vi "SetTrigger.vi"(8 "error in (no error)":errorcluster, 10 "Settings.Trigger":T1, 11 "ThorLabsCsCamera in":refnum<class "ThorLabsCsCamera.lvclass">) -> (0 "error out":errorcluster, 2 "Settings.Trigger  out":T1, 3 "ThorLabsCsCamera out":refnum<class "ThorLabsCsCamera.lvclass">)   [LabVIEW 2020, in "ThorLabsCsCamera.lvclass"]
uses:
  ThorLabsCsCamera.lvclass
  OnOffTypeDef.ctl
  ThorLabsCsCamera.lvclass/ThorLabsCsCamera.ctl
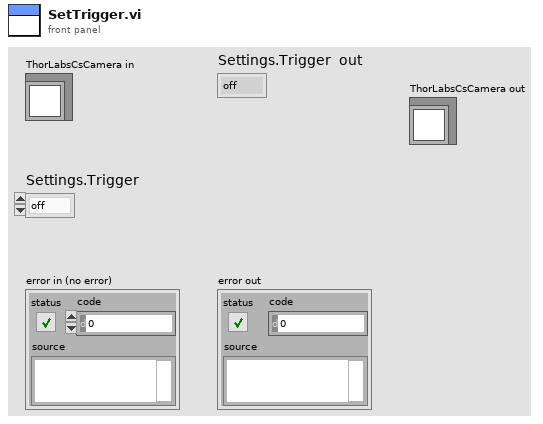
[diagram p1: front panel]
types:
  T1 = typedef "OnOffTypeDef.ctl" = enum16{"off", "on"}
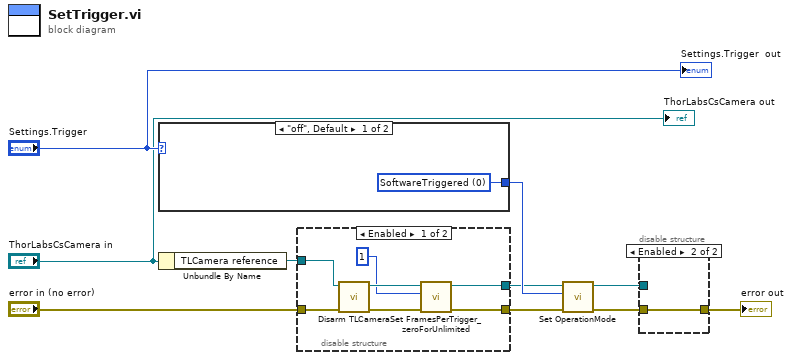
[diagram p0: block diagram]
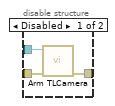
[diagram p2: hidden frame]
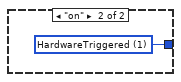
[diagram p4: hidden frame]
diagram:
  n1 = case shown="\"off\", Default" "Settings.Trigger" {
    tunnel: [w11 w12] -> w10
    frame "off", Default {
      w11 = 0 items=["SoftwareTriggered", "HardwareTriggered", "Bulb", "Reserved1", "Reserved2"] ("OperationMode")
    }
    frame "on" {
      w12 = 1 items=["SoftwareTriggered", "HardwareTriggered", "Bulb", "Reserved1", "Reserved2"] ("OperationMode")
    }
  }
  n2 = Unbundle By Name("ThorLabsCsCamera in") -> ("TLCamera reference"=w7:refnum<k24>)
  n3 = disable-structure shown="Enabled" {
    disable-tunnel: w7 -> [w19 w20]
    disable-tunnel: [w17 w20] -> w6
    disable-tunnel: "error in (no error)" -> [w16 w21]
    disable-tunnel: [w14 w21] -> w3
    frame Enabled {
      n4 = call "Disarm TLCamera.vi"("error in (no error)"=w16, "TLCamera reference"=w19) -> ("error out"=w15:errorcluster, "TLCamera reference out"=w18:refnum<k24>)  [unwired: 8 in]
      n5 = call "Set FramesPerTrigger_zeroForUnlimited.vi"("error in (no error)"=w15, "FramesPerTrigger_zeroForUnlimited"=u32 1, "TLCamera reference in"=w18) -> ("error out"=w14:errorcluster, "TLCamera reference out"=w17:refnum<k24>)  [unwired: 7 in]
    }
    frame Disabled {
    }
  }
  n6 = call "Set OperationMode.vi"("error in (no error)"=w3, "OperationMode"=w10, "TLCamera reference in"=w6) -> ("error out"=w2:errorcluster, "TLCamera reference out"=w5:refnum<k24>)  [unwired: 7 in]
  n7 = disable-structure shown="Enabled" {
    disable-tunnel: w5 -> [w24 _]
    disable-tunnel: w2 -> [w23 w25]
    disable-tunnel: [w22 w25] -> w1
    frame Disabled {
      n8 = call "Arm TLCamera.vi"("error in (no error)"=w23, "TLCamera reference"=w24) -> ("error out"=w22:errorcluster)  [unwired: 8 in, 1 out]
    }
    frame Enabled {
    }
  }
  "error out" <- w1
  "Settings.Trigger  out" <- "Settings.Trigger"
  "ThorLabsCsCamera out" <- "ThorLabsCsCamera in"
